vi "ReadMSO.vi"(0 "object in":refnum<class "AD2_SDK.lvclass">, 5 "error in (no error)":errorcluster) -> (14 "object out":refnum<class "AD2_SDK.lvclass">, 16 "Channels array":waveform(dbl)[](array[waveform]), 19 "error out":errorcluster)   [LabVIEW 2019, in "AD2_SDK.lvclass"]
uses:
  AD2_SDK.lvclass
  AD2_MSO_SDK_class/AD2_MSO_SDK.lvclass
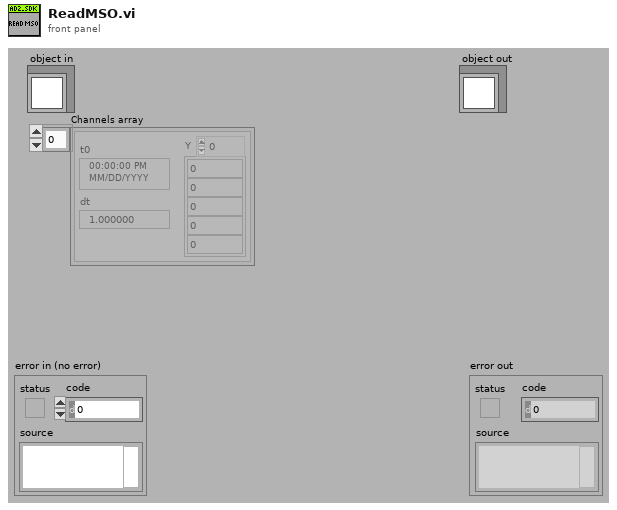
[diagram p1: front panel]
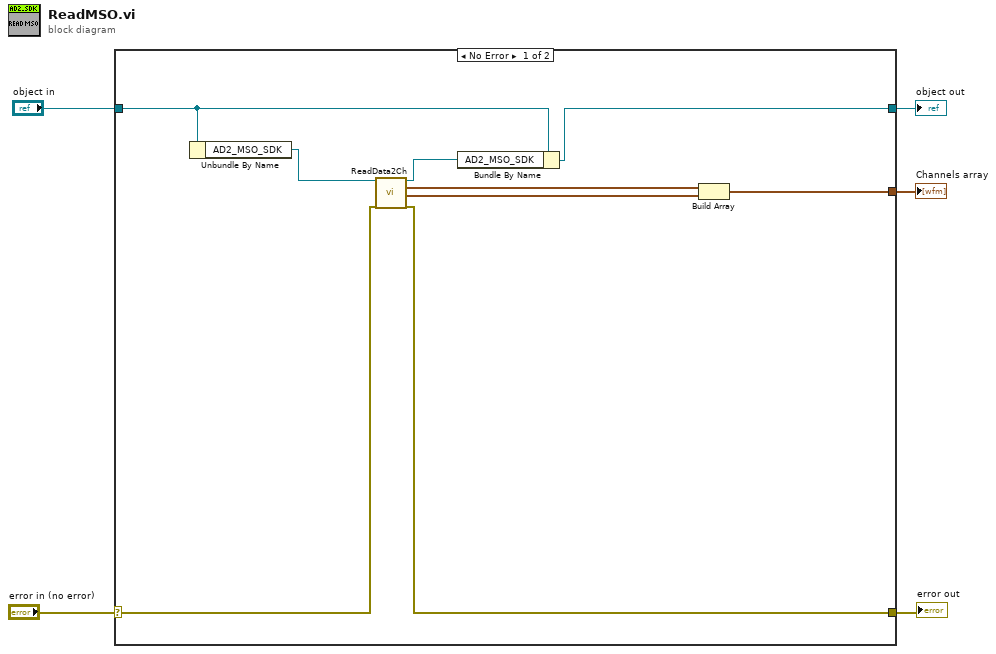
[diagram p0: block diagram]
diagram:
  n1 = case shown="No Error" "error in (no error)" {
    selector: "error in (no error)" -> [w10 w16]
    tunnel: [w9 w16] -> w4
    tunnel: [w13 w15] -> w2
    tunnel: "object in" -> [w12 w15]
    tunnel: [w6 _] -> w1
    frame No Error {
      n2 = Unbundle By Name(w12) -> ("AD2_MSO_SDK"=w14:refnum<class "AD2_MSO_SDK.lvclass">)
      n3 = call-dynamic "ReadData2Ch.vi"("object in"=w14, "error in (no error)"=w10) -> ("object out"=w11:refnum<class "AD2_MSO_SDK.lvclass">, "Ch1"=w8:waveform(dbl), "CH2"=w7:waveform(dbl), "error out"=w9:errorcluster)  [unwired: 14 in]
      n4 = Bundle By Name(cluster=w12, "AD2_MSO_SDK"=w11) -> (w13:refnum<class "AD2_SDK.lvclass">)
      n5 = Build Array(w8, w7) -> (w6:waveform(dbl)[])
    }
    frame Error {
    }
  }
  "error out" <- w4
  "object out" <- w2
  "Channels array" <- w1
